vi "remote.Write Session.TCPIP.ConnectTimeoutPerIP.vi"(8 "error in (no error)":errorcluster, 10 "Session.TCPIP.ConnectTimeoutPerIP":dbl, 11 "SLSC Remote in":refnum<class "SLSC Interface.lvclass">) -> (0 "error out":errorcluster, 3 "SLSC Remote out":refnum<class "SLSC Interface.lvclass">)   [LabVIEW 2016, in "SLSC Interfaces.lvlib" / "SLSC Interface.lvclass"]
uses:
  SLSC Interface Class/SLSC Interface.lvclass
  <vilib>/NI/JSON Support for LabVIEW/JSON Data Classes/JSON Helper/JSON Helper.lvclass
  <vilib>/NI/JSON Support for LabVIEW/JSON Data Classes/JSON Numeric/New JSON Numeric.vi
  <vilib>/NI/JSON Support for LabVIEW/JSON Data Classes/JSON Numeric/JSON Numeric.lvclass
  C:/Program Files (x86)/National Instruments/LabVIEW 2016/vi.lib/NI/JSON Support for LabVIEW/JSON Data Classes/JSON Basic Type/JSON Literal.lvclass
  C:/Program Files (x86)/National Instruments/LabVIEW 2016/vi.lib/NI/JSON Support for LabVIEW/JSON Data Classes/JSON Datatype/JSON Null.lvclass
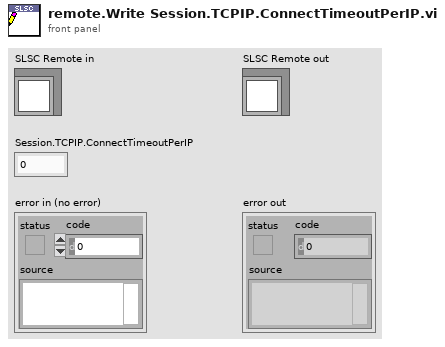
[diagram p1: front panel]
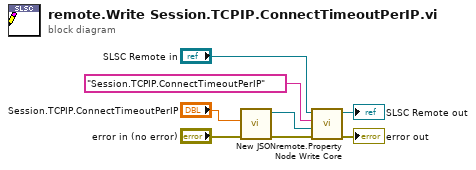
[diagram p0: block diagram]
diagram:
  n1 = call-poly <vilib>:"New JSON.vi"("error in (no error)"="error in (no error)", "value"="Session.TCPIP.ConnectTimeoutPerIP") -> ("error out"=w4:errorcluster, "JSON String out"=w3:refnum<class "JSON Numeric.lvclass">)  [unwired: 8 in]
  n2 = call "remote.Property Node Write Core.vi"("error in (no error)"=w4, "value"=w3, "property"="Session.TCPIP.ConnectTimeoutPerIP", "SLSC Remote in"="SLSC Remote in") -> ("error out"=→"error out":errorcluster, "SLSC Remote out"=→"SLSC Remote out":refnum<class "SLSC Interface.lvclass">)  [unwired: 6 in]
